vi "NFILE1.vi"(0 "Frekvence":dbl=10.0 format="%0.2p", 1 "Amplituda":dbl=1.0 format="%0.2p", 2 "Amplituda sumu":T2, 3 "Fáze":dbl, 4 "Offset":dbl format="%0.2p", 5 "Sirka okna (ms)":i32(listbox), 7 "Fvz":T1=1000.0) -> (16 "Waveform Graph":waveform(dbl)(graph))   [LabVIEW 2019]
uses:
  Control 3.ctl
  Control 1.ctl
  <vilib>/measure/NI_MABase.lvlib
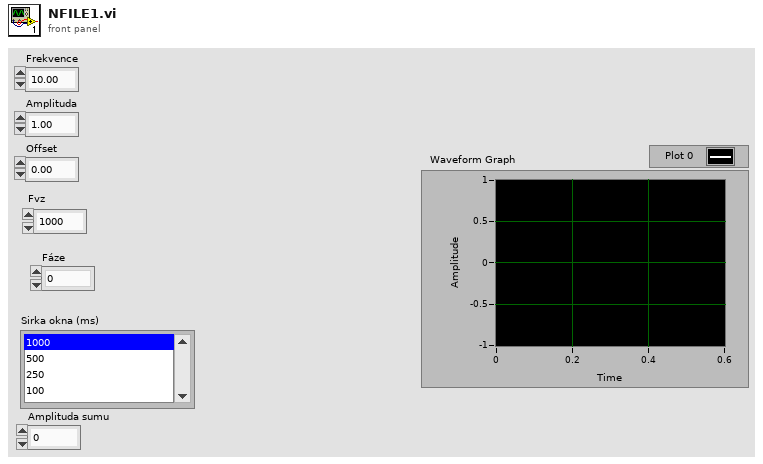
[diagram p1: front panel]
types:
  T1 = typedef "Control 1.ctl" = dbl
  T2 = typedef "Control 3.ctl" = dbl
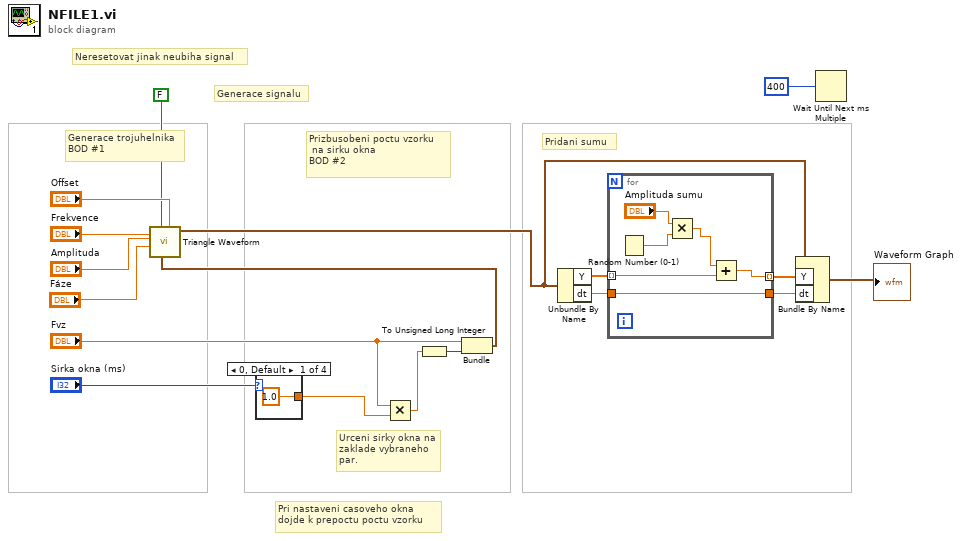
[diagram p0: block diagram]
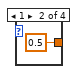
[diagram p2: hidden frame]
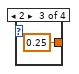
[diagram p3: hidden frame]
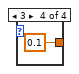
[diagram p4: hidden frame]
diagram:
  # "Generace signalu"
  # "Pri nastaveni casoveho okna \ndojde k prepoctu poctu vzorku"
  # "Pridani sumu"
  # "Neresetovat jinak neubiha signal"
  # "Urceni sirky okna na\nzaklade vybraneho par."
  # "Prizbusobeni poctu vzorku\n na sirku okna\nBOD #2"
  # "Generace trojuhelnika\nBOD #1"
  n1 = case shown="0, Default" "Sirka okna (ms)" {
    tunnel: [1.0 ("X Scale.Range:Maximum") 0.5 ("X Scale.Range:Maximum") 0.25 ("X Scale.Range:Maximum") 0.1 ("X Scale.Range:Maximum")] -> w14
    frame 0, Default {
    }
    frame 1 {
    }
    frame 2 {
    }
    frame 3 {
    }
  }
  n2 = Multiply(x="Fvz", y=w14) -> (x*y=w10:T1)
  n3 = To Unsigned Long Integer(number=w10) -> (unsigned 32bit integer=w11:u32)
  n4 = Bundle("Fvz"="Fvz", w11) -> (w12:cluster{"Fvz":T1, u32})  [unwired: 1 in]
  n5 = call <vilib>:"Triangle Waveform.vi"("offset"="Offset", "sampling info"=w12, "reset signal"=FALSE, "phase"="Fáze", "amplitude"="Amplituda", "frequency"="Frekvence") -> ("signal out"=w4:waveform(dbl))  [unwired: 4 in, 1 out]
  n6 = Unbundle By Name(w4) -> ("Y"=w8:dbl[], "dt"=w6:dbl)
  n7 = for {
    tunnel: w8 -> [w25] mode=indexing
    tunnel: [w24] -> w7 mode=indexing
    tunnel: w6 -> [w23]
    tunnel: [w23] -> w5
    n8 = Random Number (0-1)() -> (number: 0 to 1=w27:dbl)
    n9 = Multiply(x="Amplituda sumu", y=w27) -> (x*y=w26:T2)
    n10 = Add(x=w26, y=w25) -> (x+y=w24:T2)
  }
  n11 = Bundle By Name(cluster=w4, "Y"=w7, "dt"=w5) -> (→"Waveform Graph":waveform(dbl))
  n12 = Wait Until Next ms Multiple(millisecond multiple=u32 400) -> ()  [unwired: 1 out]
